vi "Command_Curvature_Distance.vi"(7 "Startup":bool, 8 "Timeout":dbl, 9 "Linear Speed":dbl, 10 "Distance(feet)":dbl, 11 "Radius(in)":dbl) -> (1 "Curvature Output":dbl, 2 "Linear Speed Output":dbl, 4 "Reint":bool, 6 "Completed":bool)   [LabVIEW 2019]
uses:
  Auto Utilities/Command_Execution_State.ctl
  Subsystems/Sensing/Sensor_Values.vi
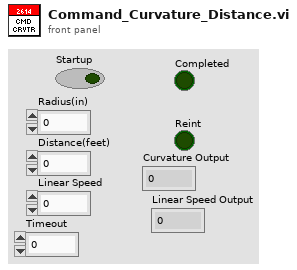
[diagram p1: front panel]
types:
  T1 = typedef "Command_Execution_State.ctl" = enum16{"Initialize", "Execute", "Finish"}
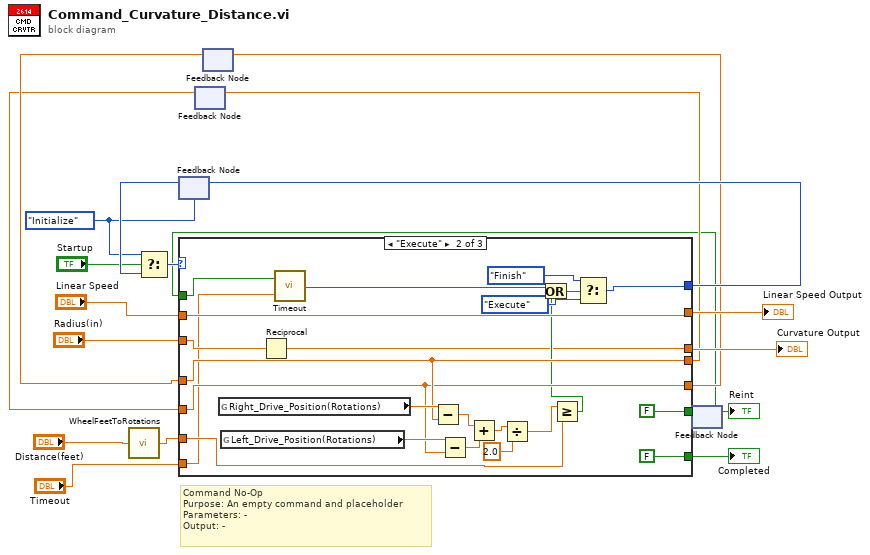
[diagram p0: block diagram]
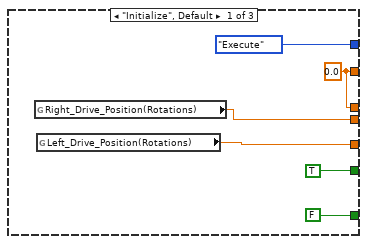
[diagram p2: hidden frame]
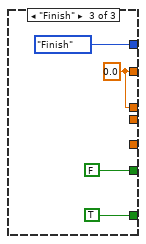
[diagram p3: hidden frame]
diagram:
  w14 = Command_Execution_State."Initialize" ("Play State")
  # "Command No-Op\nPurpose: An empty command and placeholder\nParameters: -\nOutput: -"
  n1 = call "WheelFeetToRotations.vi"("feet"="Distance(feet)") -> ("rotations"=w5:dbl)  [unwired: 4 in]
  n2 = feedback #1(w14) -> (w17:T1)
  n3 = Select(t=w14, s="Startup", f=w17) -> (s? t:f=w19:T1)
  n4 = feedback #2() -> (w6:dbl)  [unwired: 1 in]
  n5 = feedback #3() -> (w7:dbl)  [unwired: 1 in]
  n6 = feedback #4() -> (w2:bool)  [unwired: 1 in]
  "Reint" <- w2
  n7 = case shown="\"Execute\"" w19 {
    tunnel: [Command_Execution_State."Execute" ("Play State") w44 Command_Execution_State."Finish" ("Play State")] -> w18
    tunnel: [FALSE FALSE TRUE] -> w16
    tunnel: [TRUE FALSE FALSE] -> w3
    tunnel: "Radius(in)" -> [_ w46 _]
    tunnel: [w22 w26 w49] -> w12
    tunnel: "Linear Speed" -> [_ w45 _]
    tunnel: [w22 w45 w49] -> w10
    tunnel: [w21 w40 _] -> w9
    tunnel: [w20 w38 _] -> w8
    tunnel: w7 -> [_ w40 _]
    tunnel: w6 -> [_ w38 _]
    tunnel: w5 -> [_ w32 _]
    tunnel: w2 -> [_ w28 _]
    tunnel: "Timeout" -> [_ w27 _]
    frame "Initialize", Default {
      w22 = 0.0 ("Linear Speed")
      n8 = global read "Sensor_Values.vi" "Right_Drive_Position(Rotations)"() -> (w21:dbl)
      n9 = global read "Sensor_Values.vi" "Left_Drive_Position(Rotations)"() -> (w20:dbl)
    }
    frame "Execute" {
      n10 = global read "Sensor_Values.vi" "Right_Drive_Position(Rotations)"() -> (w41:dbl)
      n11 = global read "Sensor_Values.vi" "Left_Drive_Position(Rotations)"() -> (w39:dbl)
      n12 = Reciprocal(x=w46) -> (1/x=w26:dbl)
      n13 = call "Timeout.vi"("Timeout"=w27, "Initialize"=w28) -> ("Timed Out?"=w29:bool)
      n14 = Subtract(x=w41, y=w40) -> (x-y=w37:dbl)
      n15 = Subtract(x=w39, y=w38) -> (x-y=w36:dbl)
      n16 = Add(x=w37, y=w36) -> (x+y=w35:dbl)
      n17 = Divide(x=w35, y=2.0) -> (x/y=w33:dbl)
      n18 = Greater Or Equal?(x=w33, y=w32) -> (x >= y?=w30:bool)
      n19 = Or(x=w29, y=w30) -> (x .or. y?=w31:bool)
      n20 = Select(t=Command_Execution_State."Finish" ("Play State"), s=w31, f=Command_Execution_State."Execute" ("Play State")) -> (s? t:f=w44:T1)
    }
    frame "Finish" {
      w49 = 0.0 ("Linear Speed")
    }
  }
  "Completed" <- w16
  "Curvature Output" <- w12
  "Linear Speed Output" <- w10
  n21 = feedback-in #1(w18) -> ()
  n22 = feedback-in #2(w9) -> ()
  n23 = feedback-in #3(w8) -> ()
  n24 = feedback-in #4(w3) -> ()
